vi "Add Tree.vi"(7 "Parent ID":string, 8 "Error In":errorcluster, 10 "Child ID":string, 11 "Tree Manager":T1) -> (0 "Error Out":errorcluster, 3 "Tree Manager":T1)   [LabVIEW 2016, in "Tree Manager.lvclass"]
doc: "Add a Tree under a specific Parent. Both the added Tree and the Parent have to exist in the Tree Manager.\n\nIf the Tree has a parent before the new Parent replaces it. This means this method can also be used to perform a move operation."
uses:
  Tree Manager.lvclass
  Typedefs/Session Handle.ctl
  Tree Manager.lvclass/Tree Manager.ctl
  Private/Build Missing Tree Error.vi
  Private/Build Empty ID Error.vi
  Private/Add to Parent Priv.vi
  Private/Remove from Parent Priv.vi
  <vilib>/Utility/error.llb/Error Cluster From Error Code.vi
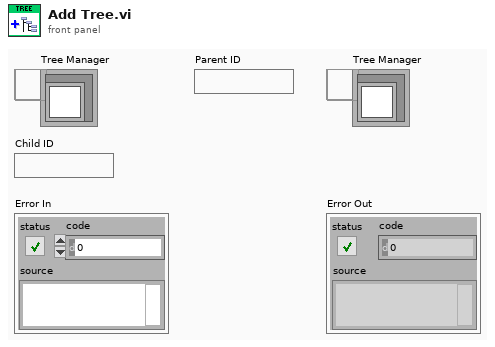
[diagram p1: front panel]
types:
  T1 = typedef "Tree Manager.lvclass/Session Handle.ctl" = refnum<data-value>
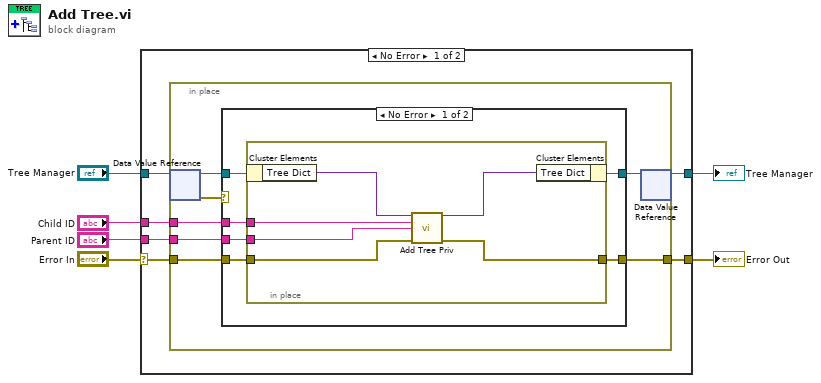
[diagram p0: block diagram]
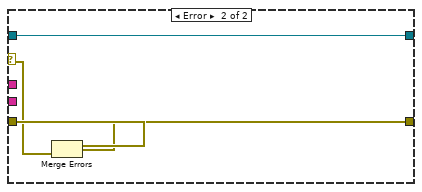
[diagram p2: hidden frame]
diagram:
  n1 = case shown="No Error" "Error In" {
    selector: "Error In" -> [w10 w36]
    tunnel: "Tree Manager" -> [w12 w37]
    tunnel: [w11 w37] -> w5
    tunnel: [w9 w36] -> w3
    tunnel: "Child ID" -> [w8 _]
    tunnel: "Parent ID" -> [w7 _]
    frame No Error {
      n2 = in-place {
        in-place-border: w10 -> [w15]
        in-place-border: [w18] -> w9
        in-place-border: w8 -> [w14]
        in-place-border: w7 -> [w13]
        n3 = in-place-dvr #1(w12) -> (w19:refnum<class "Tree Manager.lvclass">, w16:errorcluster)
        n4 = case shown="No Error" w16 {
          selector: w16 -> [_ w34]
          tunnel: w19 -> [w25 w32]
          tunnel: [w24 w33] -> w18
          tunnel: [w23 w32] -> w17
          tunnel: w15 -> [w22 w35]
          tunnel: w14 -> [w21 _]
          tunnel: w13 -> [w20 _]
          frame No Error {
            n5 = in-place {
              in-place-border: [w29] -> w24
              in-place-border: w22 -> [w28]
              in-place-border: w21 -> [w27]
              in-place-border: w20 -> [w26]
              n6 = in-place-cluster #2(w25) -> ("Tree Dict"=w31:variant)
              n7 = call "Add Tree Priv.vi"("Tree Dictionary In"=w31, "Unique ID"=w27, "Parent ID"=w26, "Error In"=w28) -> ("Tree Dictionary Out"=w30:variant, "Error Out"=w29:errorcluster)  [unwired: 10 in]
              n8 = in-place-cluster #2("Tree Dict"=w30) -> (w23:refnum<class "Tree Manager.lvclass">)
            }
          }
          frame Error {
            n9 = Merge Errors(w35, w34) -> (w33:errorcluster)
          }
        }
        n10 = in-place-dvr #1(w17) -> (w11:T1)  [unwired: 1 out]
      }
    }
    frame Error {
    }
  }
  "Tree Manager" <- w5
  "Error Out" <- w3
